vi "initializeDisplay.vi"(8 "error in (no error)":errorcluster, 9 "uiControlsMgr.lvclass":refnum<class "uiControlsMgr.lvclass">) -> (0 "error out":errorcluster, 3 "TextDisplay Class out":refnum<class "TextDisplay Class.lvclass">)   [LabVIEW 2020, in "TextDisplay Class.lvclass"]
uses:
  TextDisplay Class.lvclass
  uiControlsMgr/uiControlsMgr.lvclass
  TextDisplay Class.lvclass/TextDisplay Class.ctl
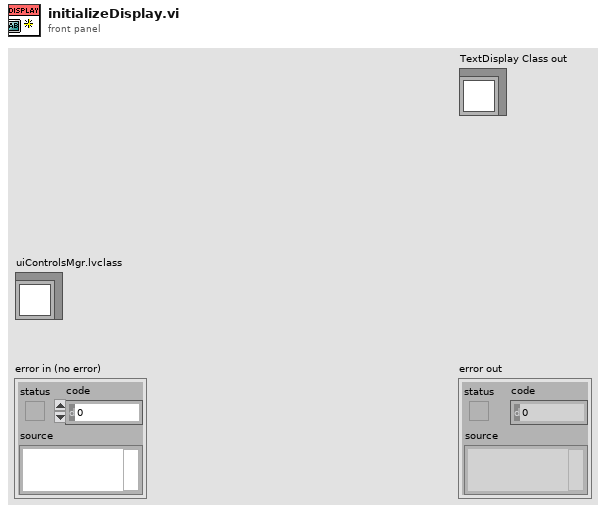
[diagram p1: front panel]
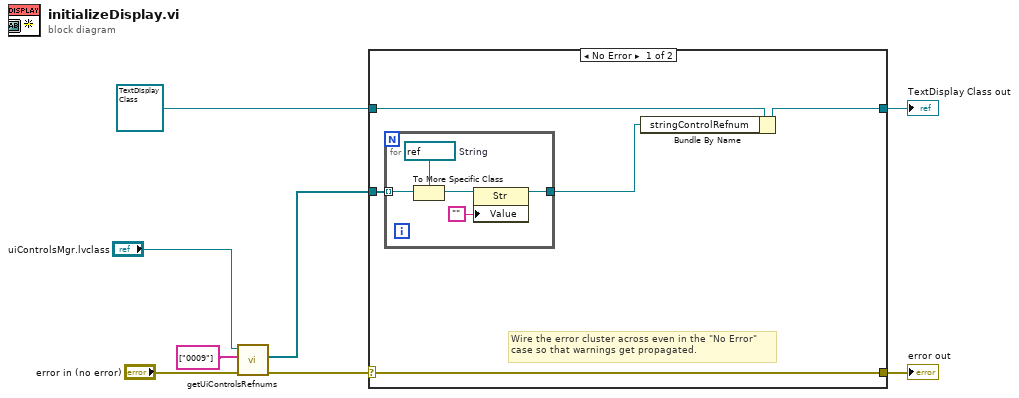
[diagram p0: block diagram]
diagram:
  n1 = call "getUiControlsRefnums.vi"("error in (no error)"="error in (no error)", "Control Indexes"=string[] ["0009"], "uiControlsMgr in"="uiControlsMgr.lvclass") -> ("error out"=w2:errorcluster, "Control Refnums"=w1:refnum<vi>[])  [unwired: 6 in, 1 out]
  n2 = case shown="No Error" w2 {
    selector: w2 -> [w12 w20]
    tunnel: [w12 w20] -> w8
    tunnel: [w11 w19] -> w6
    tunnel: refnum<class "TextDisplay Class.lvclass"> refnum ("TextDisplay Class in") -> [w13 w19]
    tunnel: w1 -> [w10 _]
    frame No Error {
      # "Wire the error cluster across even in the \"No Error\"\ncase so that warnings get propagated."
      n3 = for {
        tunnel: w10 -> [w14] mode=indexing
        tunnel: [w18] -> w9
        w16 = refnum<vi> refnum  # String
        n4 = To More Specific Class(target class=w16, reference=w14) -> (specific class reference=w15:refnum<vi>)  [unwired: 1 in, 1 out]
        n5 = property class="Str"(reference=w15, "Value"="") -> (reference out=w18:refnum<vi>)  [unwired: 1 in, 1 out]
      }
      n6 = Bundle By Name(cluster=w13, "stringControlRefnum"=w9) -> (w11:refnum<class "TextDisplay Class.lvclass">)
    }
    frame Error {
    }
  }
  "error out" <- w8
  "TextDisplay Class out" <- w6
